vi "HW_Setup.vi"(6 "Close port? (T)":bool=TRUE, 8 "error in":errorcluster, 9 "Traget FPS":i32=80, 11 "VISA resource name in":refnum<visa-resource-name>="ASRL3::INSTR") -> (0 "FPS status":i32=80, 1 "Instrument OK?":bool=TRUE, 2 "Data flow controls":T1, 3 "VISA resource name out":refnum<visa-resource-name>="ASRL3::INSTR", 4 "Version information":string, 5 "Sensor board size":string, 7 "error out":errorcluster, 10 "Sync mode status":string)   [LabVIEW 2018, in "Tracker.lvlib"]
uses:
  Tracker.lvlib
  Controls/CTL_Data_flow_control_cluster.ctl
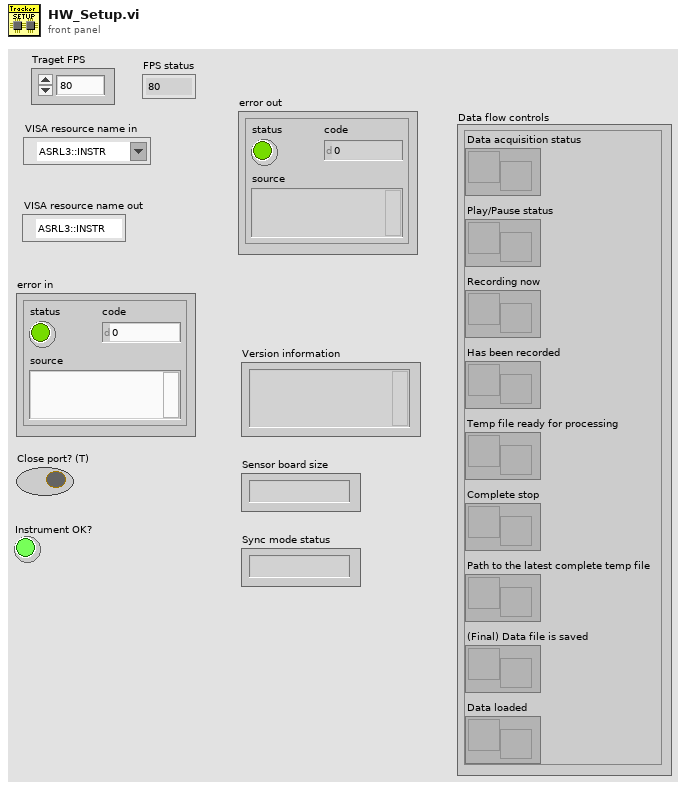
[diagram p1: front panel]
types:
  T1 = typedef "Tracker.lvlib/CTL_Data_flow_control_cluster.ctl" = cluster{"Data acquisition status":refnum<notifier>, "Play/Pause status":refnum<notifier>, "Complete stop":refnum<notifier>, "Temp file ready for processing":refnum<notifier>, "Has been recorded":refnum<notifier>, "Recording now":refnum<notifier>, "Path to the latest complete temp file":refnum<notifier>, "(Final) Data file is saved":refnum<notifier>, "Data loaded":refnum<notifier>}
  T2 = cluster{"notifier out":refnum<notifier>, "notifier out":refnum<notifier>, "notifier out":refnum<notifier>, "notifier out":refnum<notifier>, "notifier out":refnum<notifier>, "notifier out":refnum<notifier>, "notifier out":refnum<notifier>, "notifier out":refnum<notifier>, "notifier out":refnum<notifier>}
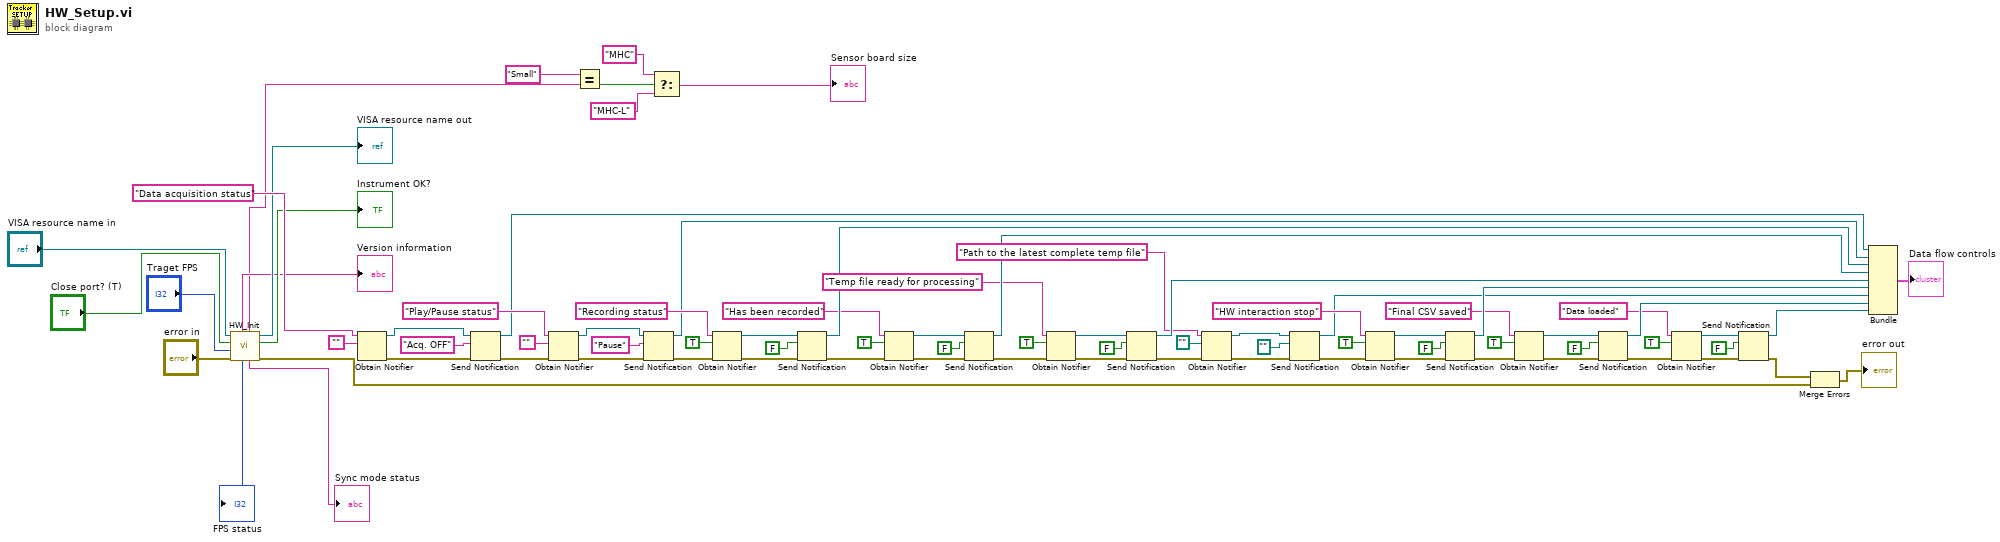
[diagram p0: block diagram]
diagram:
  n1 = call "HW_Init.vi"("error in"="error in", "Traget FPS"="Traget FPS", "Close port? (T)"="Close port? (T)", "VISA resource name"="VISA resource name in") -> ("error out"=w8:errorcluster, "Instrument OK?"=→"Instrument OK?":bool, "VISA resource name out"=→"VISA resource name out":refnum<visa-resource-name>, "Sync mode status"=→"Sync mode status":string, "Sensor board size"=w10:string, "FPS status"=→"FPS status":i32, "Version information"=→"Version information":string)  [unwired: 1 out]
  n2 = Obtain Notifier(name (unnamed)="Data acquisition status", notification data type="") -> (notifier out=w77:refnum<notifier>, error out=w75:errorcluster)  [unwired: 2 in, 1 out]
  n3 = Send Notification(notification="Acq. OFF", notifier=w77, error in (no error)=w75) -> (notifier out=w64:refnum<notifier>, error out=w69:errorcluster)
  n4 = Obtain Notifier(name (unnamed)="Play/Pause status", notification data type="", error in (no error)=w69) -> (notifier out=w72:refnum<notifier>, error out=w74:errorcluster)  [unwired: 1 in, 1 out]
  n5 = Equal?(x="Small", y=w10) -> (x = y?=w5:bool)
  n6 = Send Notification(notification="Pause", notifier=w72, error in (no error)=w74) -> (notifier out=w63:refnum<notifier>, error out=w65:errorcluster)
  n7 = Select(t="MHC" ("x"), s=w5, f="MHC-L") -> (s? t:f=→"Sensor board size":string)
  n8 = Obtain Notifier(name (unnamed)="Recording status", notification data type=TRUE, error in (no error)=w65) -> (notifier out=w67:refnum<notifier>, error out=w66:errorcluster)  [unwired: 1 in, 1 out]
  n9 = Send Notification(notification=FALSE, notifier=w67, error in (no error)=w66) -> (notifier out=w62:refnum<notifier>, error out=w54:errorcluster)
  n10 = Obtain Notifier(name (unnamed)="Has been recorded", notification data type=TRUE, error in (no error)=w54) -> (notifier out=w52:refnum<notifier>, error out=w55:errorcluster)  [unwired: 1 in, 1 out]
  n11 = Send Notification(notification=FALSE, notifier=w52, error in (no error)=w55) -> (notifier out=w51:refnum<notifier>, error out=w50:errorcluster)
  n12 = Obtain Notifier(name (unnamed)="Temp file ready for processing", notification data type=TRUE, error in (no error)=w50) -> (notifier out=w47:refnum<notifier>, error out=w49:errorcluster)  [unwired: 1 in, 1 out]
  n13 = Send Notification(notification=FALSE, notifier=w47, error in (no error)=w49) -> (notifier out=w46:refnum<notifier>, error out=w35:errorcluster)
  n14 = Obtain Notifier(name (unnamed)="Path to the latest complete temp file", notification data type=path "", error in (no error)=w35) -> (notifier out=w31:refnum<notifier>, error out=w33:errorcluster)  [unwired: 1 in, 1 out]
  n15 = Send Notification(notification=path "", notifier=w31, error in (no error)=w33) -> (notifier out=w29:refnum<notifier>, error out=w32:errorcluster)
  n16 = Obtain Notifier(name (unnamed)="HW interaction stop", notification data type=TRUE, error in (no error)=w32) -> (notifier out=w42:refnum<notifier>, error out=w43:errorcluster)  [unwired: 1 in, 1 out]
  n17 = Send Notification(notification=FALSE, notifier=w42, error in (no error)=w43) -> (notifier out=w30:refnum<notifier>, error out=w24:errorcluster)
  n18 = Obtain Notifier(name (unnamed)="Final CSV saved", notification data type=TRUE, error in (no error)=w24) -> (notifier out=w21:refnum<notifier>, error out=w22:errorcluster)  [unwired: 1 in, 1 out]
  n19 = Send Notification(notification=FALSE, notifier=w21, error in (no error)=w22) -> (notifier out=w19:refnum<notifier>, error out=w18:errorcluster)
  n20 = Obtain Notifier(name (unnamed)="Data loaded", notification data type=TRUE, error in (no error)=w18) -> (notifier out=w16:refnum<notifier>, error out=w17:errorcluster)  [unwired: 1 in, 1 out]
  n21 = Send Notification(notification=FALSE, notifier=w16, error in (no error)=w17) -> (notifier out=w15:refnum<notifier>, error out=w7:errorcluster)
  n22 = Merge Errors(w7, w8) -> (→"error out":errorcluster)
  n23 = Bundle("notifier out"=w64, "notifier out"=w63, "notifier out"=w62, "notifier out"=w51, "notifier out"=w46, "notifier out"=w30, "notifier out"=w29, "notifier out"=w19, "notifier out"=w15) -> (→"Data flow controls":T2)  [unwired: 1 in]
